vi "SetRef.vi"(8 "error in (no error)":errorcluster, 10 "ref":u64, 11 "ByRefClass in":refnum<class "ClassByRef.lvclass">) -> (0 "error out":errorcluster, 3 "ByRefClass out":refnum<class "ClassByRef.lvclass">)   [LabVIEW 2021, in "ClassUtilities.lvlib" / "ClassByRef.lvclass"]
uses:
  ClassByRef.lvclass
  ClassByRef.lvclass/ClassByRef.ctl
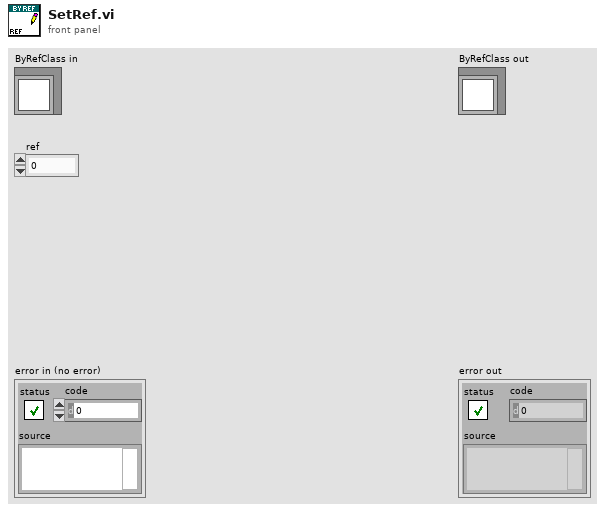
[diagram p1: front panel]
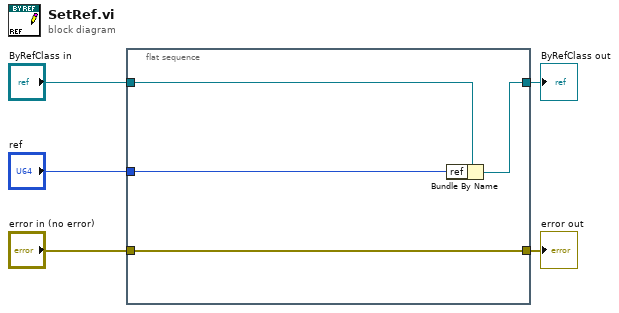
[diagram p0: block diagram]
diagram:
  n1 = flat-sequence {
    tunnel: "ByRefClass in" -> [w9]
    tunnel: [w8] -> w4
    tunnel: "ref" -> [w7]
    tunnel: "error in (no error)" -> [w6]
    tunnel: [w6] -> w1
    frame #0 {
      n2 = Bundle By Name(cluster=w9, "ref"=w7) -> (w8:refnum<class "ClassByRef.lvclass">)
    }
  }
  "error out" <- w1
  "ByRefClass out" <- w4
